vi "Read Text.vi"(6 "timeout ms (5000)":i32=5000, 8 "error in":errorcluster, 9 "RawSocket Handler in":refnum<class "RawSocket Handler.lvclass">) -> (1 "String":string, 2 "error out":errorcluster, 3 "RawSocket Handler out":refnum<class "RawSocket Handler.lvclass">)   [LabVIEW 2020, in "wamplv.lvlib" / "RawSocket Handler.lvclass"]
uses:
  RawSocket Handler.lvclass
  RawSocket Handler.lvclass/RawSocket Handler.ctl
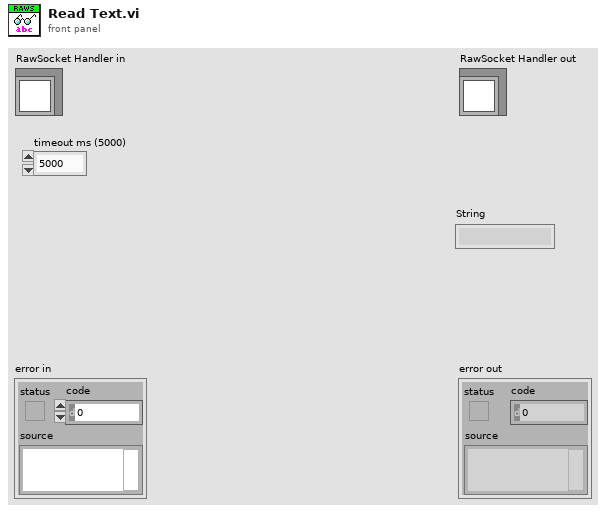
[diagram p1: front panel]
types:
  T1 = typedef "wamplv.lvlib/RawSocket Handler.lvclass/Message Type.ctl" = enum8{"Regular WAMP message", "PING", "PONG"}
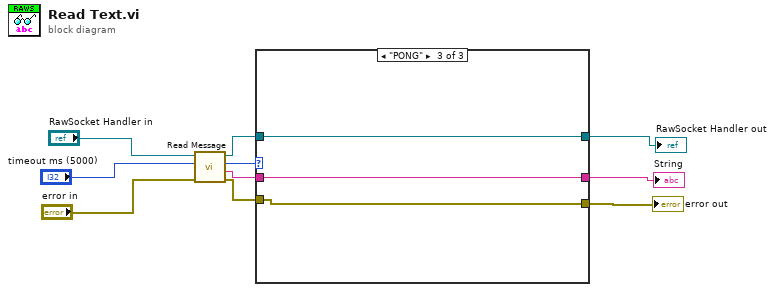
[diagram p0: block diagram]
diagram:
  n1 = call-dynamic "Read Message.vi"("error in"="error in", "timeout ms (5000)"="timeout ms (5000)", "RawSocket Handler in"="RawSocket Handler in") -> ("error out"=w4:errorcluster, "Message data"=w6:string, "Message Type"=w7:T1, "RawSocket Handler out"=w1:refnum<class "RawSocket Handler.lvclass">)  [unwired: 3 in]
  n2 = case shown="\"PONG\"" w7 {
    tunnel: [w12 w15 w18] -> w5
    tunnel: w6 -> [w12 w15 w18]
    tunnel: [w13 w16 w19] -> w3
    tunnel: w4 -> [w13 w16 w19]
    tunnel: [w11 w14 w17] -> w2
    tunnel: w1 -> [w11 w14 w17]
    frame "Regular WAMP message", Default {
    }
    frame "PING" {
    }
    frame "PONG" {
    }
  }
  "error out" <- w3
  "RawSocket Handler out" <- w2
  "String" <- w5
